vi "Configure9217.vi"(7 "Channel Number":i32, 8 "error in (no error)":errorcluster, 10 "Properties":T1[](array[typedef]), 11 "IO Ref":refnum<k21>) -> (0 "error out":errorcluster, 3 "IO Ref out":refnum<k21>)   [LabVIEW 2017, in "ScanEngine.lvlib"]
uses:
  <vilib>/addons/InsightCM/Devices/Shared/Common/ScanEngine/ScanEngine.lvlib
  <vilib>/addons/InsightCM/MessageBus/Base/controls/KeyValuePair.ctl
  <resource>/objmgr/cRIO.rc
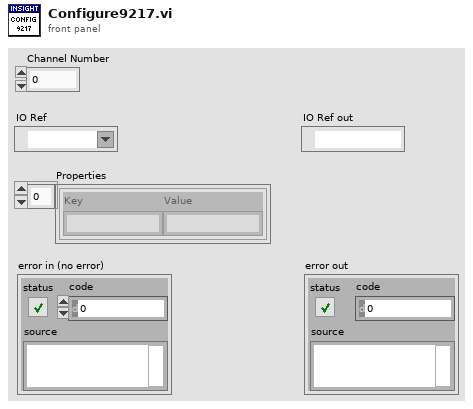
[diagram p1: front panel]
types:
  T1 = typedef "KeyValuePair.ctl" = cluster{"Key":string, "Value":string}
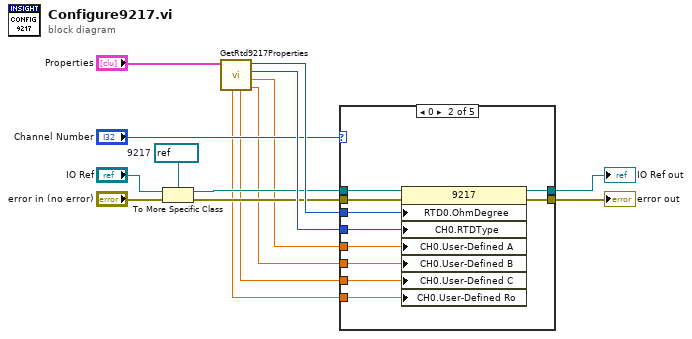
[diagram p0: block diagram]
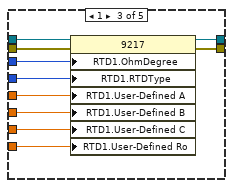
[diagram p3: hidden frame]
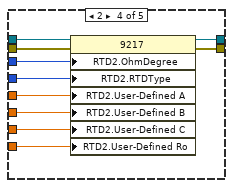
[diagram p4: hidden frame]
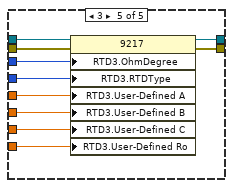
[diagram p5: hidden frame]
diagram:
  w9 = refnum<k21> refnum  # 9217
  n1 = To More Specific Class(target class=w9, reference="IO Ref", error in="error in (no error)") -> (specific class reference=w8:refnum<k21>, error out=w12:errorcluster)
  n2 = call <vilib>:"GetRtd9217Properties.vi"("Properties"="Properties") -> ("B"=w3:dbl, "A"=w4:dbl, "RTD type"=w15:u32, "RTD ohm degree range"=w14:u32, "C"=w2:dbl, "r0"=w1:dbl)  [unwired: 5 in]
  n3 = case shown="0" "Channel Number" {
    tunnel: w12 -> [w17 w24 w34 w44 w54]
    tunnel: [w17 w27 w37 w47 w57] -> w5
    tunnel: w8 -> [w16 w26 w36 w46 w56]
    tunnel: [w16 w25 w35 w45 w55] -> w11
    tunnel: w14 -> [_ w23 w33 w43 w53]
    tunnel: w15 -> [_ w22 w32 w42 w52]
    tunnel: w4 -> [_ w21 w31 w41 w51]
    tunnel: w1 -> [_ w20 w28 w38 w48]
    tunnel: w3 -> [_ w19 w30 w40 w50]
    tunnel: w2 -> [_ w18 w29 w39 w49]
    frame -1, Default {
    }
    frame 0 {
      n4 = property class="9217"(reference=w26, error in=w24, "RTD0.OhmDegree"=w23, "CH0.RTDType"=w22, "CH0.User-Defined A"=w21, "CH0.User-Defined B"=w19, "CH0.User-Defined C"=w18, "CH0.User-Defined Ro"=w20) -> (reference out=w25:refnum<k21>, error out=w27:errorcluster)
    }
    frame 1 {
      n5 = property class="9217"(reference=w36, error in=w34, "RTD1.OhmDegree"=w33, "RTD1.RTDType"=w32, "RTD1.User-Defined A"=w31, "RTD1.User-Defined B"=w30, "RTD1.User-Defined C"=w29, "RTD1.User-Defined Ro"=w28) -> (reference out=w35:refnum<k21>, error out=w37:errorcluster)
    }
    frame 2 {
      n6 = property class="9217"(reference=w46, error in=w44, "RTD2.OhmDegree"=w43, "RTD2.RTDType"=w42, "RTD2.User-Defined A"=w41, "RTD2.User-Defined B"=w40, "RTD2.User-Defined C"=w39, "RTD2.User-Defined Ro"=w38) -> (reference out=w45:refnum<k21>, error out=w47:errorcluster)
    }
    frame 3 {
      n7 = property class="9217"(reference=w56, error in=w54, "RTD3.OhmDegree"=w53, "RTD3.RTDType"=w52, "RTD3.User-Defined A"=w51, "RTD3.User-Defined B"=w50, "RTD3.User-Defined C"=w49, "RTD3.User-Defined Ro"=w48) -> (reference out=w55:refnum<k21>, error out=w57:errorcluster)
    }
  }
  "IO Ref out" <- w11
  "error out" <- w5
